vi "ChooseContour.vi"(1 "SwitchRatio":dbl, 2 "Target2":T1, 3 "Prev":T1, 4 "Target1 (preferred)":T1) -> (0 "Better":T1)   [LabVIEW 2017]
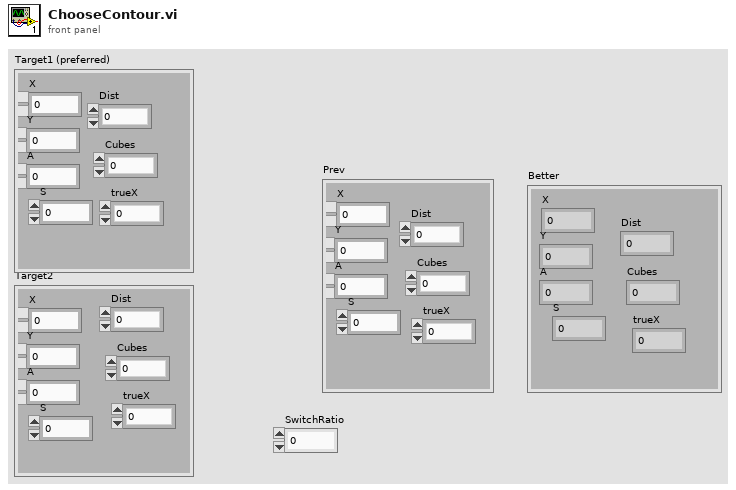
[diagram p1: front panel]
types:
  T1 = cluster{"X":dbl, "Y":dbl, "A":dbl, "S":dbl, "Dist":dbl, "Cubes":dbl, "trueX":dbl}
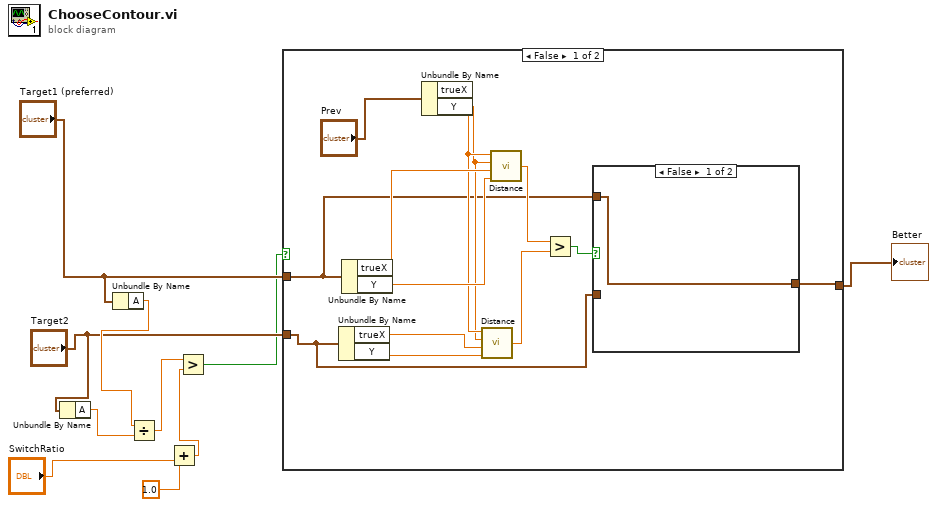
[diagram p0: block diagram]
diagram:
  n1 = Unbundle By Name("Target2") -> ("A"=w5:dbl)
  n2 = Unbundle By Name("Target1 (preferred)") -> ("A"=w7:dbl)
  n3 = Divide(x=w7, y=w5) -> (x/y=w2:dbl)
  n4 = Add(x=1.0, y="SwitchRatio") -> (x+y=w3:dbl)
  n5 = Greater?(x=w2, y=w3) -> (0:w1:bool)
  n6 = case shown="False" w1 {
    tunnel: [w12 w26] -> w10
    tunnel: "Target1 (preferred)" -> [w13 w26]
    tunnel: "Target2" -> [w14 _]
    frame False {
      n7 = Unbundle By Name(w14) -> ("trueX"=w19:dbl, "Y"=w18:dbl)
      n8 = Unbundle By Name(w13) -> ("trueX"=w23:dbl, "Y"=w22:dbl)
      n9 = Unbundle By Name("Prev") -> ("trueX"=w21:dbl, "Y"=w20:dbl)
      n10 = call "Distance.vi"("y2"=w18, "x2"=w19, "y1"=w20, "x1"=w21) -> ("dist"=w16:dbl)
      n11 = call "Distance.vi"("y2"=w22, "x2"=w23, "y1"=w20, "x1"=w21) -> ("dist"=w17:dbl)
      n12 = Greater?(x=w17, y=w16) -> (0:w15:bool)
      n13 = case shown="False" w15 {
        tunnel: w14 -> [_ w25]
        tunnel: w13 -> [w24 _]
        tunnel: [w24 w25] -> w12
        frame False {
        }
        frame True {
        }
      }
    }
    frame True {
    }
  }
  "Better" <- w10
